vi "dfd_DFXP Quantizer to Operation.vi"(1 "quantizer":T3={"source"=0, "wl"=16, "iwl"=1, "overflow mode"=enum."Wrap", "rounding mode"=enum."Truncation", "signed?"=TRUE} {"source" items=["Coef a/k"=0, "Coef b/v"=7, "Input"=1, "Output"=2, "Multiplicand"=3, "Product"=4, "Sum"=5, "Delay"=6, "Gain"=8]}) -> (0 "op params":T1={"source"=0, "is floating?"=FALSE, "o-mode"=enum."Wrap", "q-mode"=enum."Nearest", "wl"=0, "high limit"=0, "low limit"=0, "iwl"=0, "sign?"=TRUE} {"source" items=["Coef a/k"=0, "Coef b/v"=7, "Input"=1, "Output"=2, "Multiplicand"=3, "Product"=4, "Sum"=5, "Delay"=6, "Gain"=8]})   [LabVIEW 2017, in "NI_DigFilter_FXP.lvlib"]
uses:
  <vilib>/addons/Digital Filter Design/NI_DigFilter_FXP.lvlib
  <vilib>/addons/Digital Filter Design/_Objects.llb/dfd_Internal Quantization Settings.ctl
  <vilib>/addons/Digital Filter Design/_Objects.llb/dfd_Internal Quantization Srcs.ctl
  <vilib>/addons/Digital Filter Design/_Objects.llb/dfd_DFXP Operation Parameter.ctl
  <vilib>/addons/Digital Filter Design/NI_DigFilterLicensed.lvlib
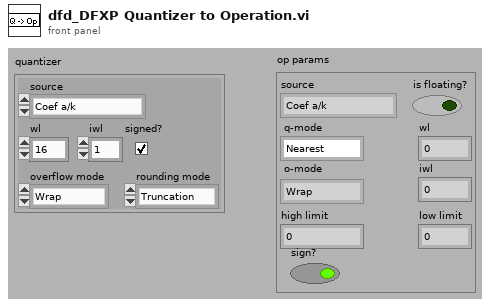
[diagram p1: front panel]
types:
  T1 = typedef "dfd_DFXP Operation Parameter.ctl" = cluster{"source":T2, "is floating?":bool, "o-mode":enum16{"Saturation", "Wrap"}, "q-mode":enum16{"Nearest", "Truncation"}, "wl":i16, "high limit":i64, "low limit":i64, "iwl":i16, "sign?":bool}
  T2 = typedef "NI_DigFilterLicensed.lvlib/dfd_Internal Quantization Srcs.ctl" = u16
  T3 = typedef "NI_DigFilterLicensed.lvlib/dfd_Internal Quantization Settings.ctl" = cluster{"source":T2, "wl":i16, "iwl":i16, "overflow mode":enum16{"Saturation", "Wrap"}, "rounding mode":enum16{"Nearest", "Truncation"}, "signed?":bool}
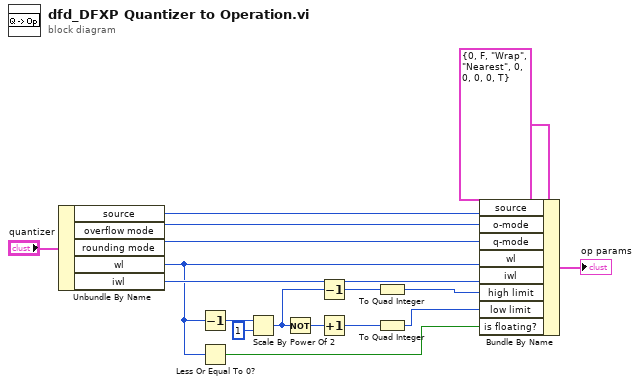
[diagram p0: block diagram]
diagram:
  n1 = Unbundle By Name("quantizer") -> ("source"=w8:T2, "overflow mode"=w9:enum16{"Saturation", "Wrap"}, "rounding mode"=w7:enum16{"Nearest", "Truncation"}, "wl"=w3:i16, "iwl"=w6:i16)
  n2 = Decrement(x=w3) -> (x-1=w12:i16)
  n3 = Less Or Equal To 0?(x=w3) -> (x <= 0?=w2:bool)
  n4 = Scale By Power Of 2(n=w12, x=u64 1) -> (x*2^n=w10:u64)
  n5 = Not(x=w10) -> (.not. x?=w11:u64)
  n6 = Decrement(x=w10) -> (x-1=w14:u64)
  n7 = Increment(x=w11) -> (x+1=w15:u64)
  n8 = To Quad Integer(1:w14) -> (0:w5:i64)
  n9 = To Quad Integer(1:w15) -> (0:w4:i64)
  n10 = Bundle By Name(cluster=T1 {"source"=0, "is floating?"=FALSE, "o-mode"=enum."Wrap", "q-mode"=enum."Nearest", "wl"=0, "high limit"=0, "low limit"=0, "iwl"=0, "sign?"=TRUE} ("op params"), "source"=w8, "o-mode"=w9, "q-mode"=w7, "wl"=w3, "iwl"=w6, "high limit"=w5, "low limit"=w4, "is floating?"=w2) -> (→"op params":T1)
